vi "Subtract DAQ Offset.vi"(8 "error in (no error)":errorcluster, 11 "Instrument.DAQ":refnum<class "Instrument.DAQ.lvclass">) -> (0 "error out":errorcluster, 3 "Instrument.DAQ out":refnum<class "Instrument.DAQ.lvclass">)   [LabVIEW 2019, in "Instrument.DAQ.lvclass"]
uses:
  Instrument.DAQ.lvclass
  Instrument.DAQ.lvclass/Instrument.DAQ.ctl
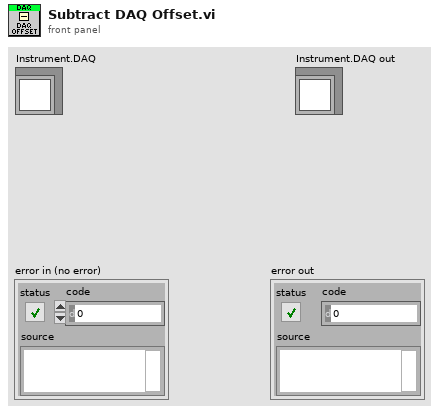
[diagram p1: front panel]
types:
  T1 = typedef "Instrument.DAQ.lvclass/Channel.Gain--Cluster--Array.ctl" = T2[]
  T2 = typedef "Instrument.DAQ.lvclass/Channel.Gain--Cluster.ctl" = cluster{"Channel":string, "Gain":dbl}
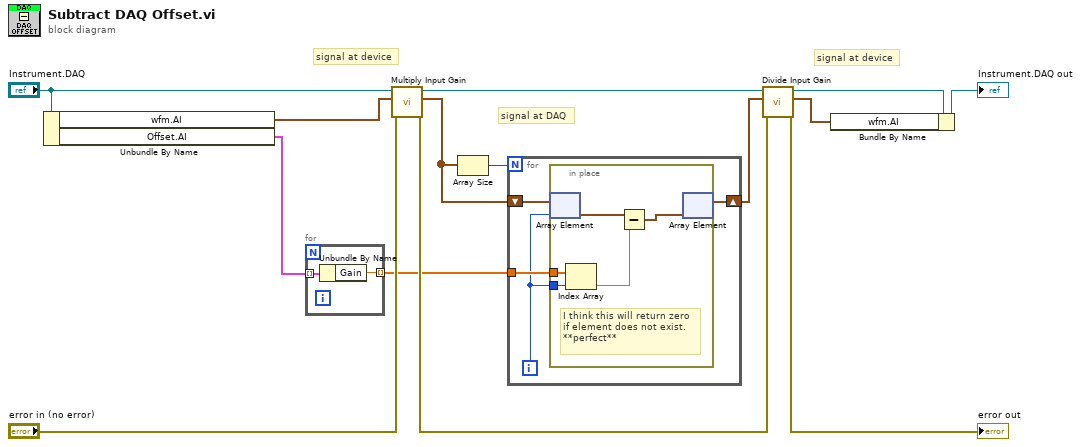
[diagram p0: block diagram]
diagram:
  # "signal at device"
  # "signal at DAQ"
  # "signal at device"
  n1 = Unbundle By Name("Instrument.DAQ") -> ("wfm.AI"=w7:waveform(dbl)[], "Offset.AI"=w4:T1)
  n2 = for {
    tunnel: w4 -> [w16] mode=indexing
    tunnel: [w15] -> w3 mode=indexing
    n3 = Unbundle By Name(w16) -> ("Gain"=w15:dbl)
  }
  n4 = call "Multiply Input Gain.vi"("error in (no error)"="error in (no error)", "WFM in"=w7, "Instrument.DAQ"="Instrument.DAQ") -> ("error out"=w10:errorcluster, "WFM out"=w5:waveform(dbl)[], "Instrument.DAQ out"=w9:refnum<class "Instrument.DAQ.lvclass">)  [unwired: 6 in]
  n5 = Array Size(array=w5) -> (size(s)=w14:i32)
  n6 = for {
    N: w14 -> [_]
    tunnel: w3 -> [w20]
    shift-right: [w17] -> w13
    shift-left: w5 -> [w18]
    i -> [w19]
    n7 = in-place {
      in-place-border: w19 -> [w25]
      in-place-border: w20 -> [w24]
      # "I think this will return zero\nif element does not exist.\n**perfect**"
      n8 = in-place-array #1(w18, w19) -> (w21:waveform(dbl))
      n9 = Index Array(array=w24, index=w25) -> (element=w23:dbl)
      n10 = Subtract(x=w21, y=w23) -> (x-y=w22:waveform(dbl))
      n11 = in-place-array #1(w22) -> (w17:waveform(dbl)[])  [unwired: 1 out]
    }
  }
  n12 = call "Divide Input Gain.vi"("error in (no error)"=w10, "WFM in"=w13, "Instrument.DAQ"=w9) -> ("error out"=→"error out":errorcluster, "WFM out"=w1:waveform(dbl)[], "Instrument.DAQ out"=w6:refnum<class "Instrument.DAQ.lvclass">)  [unwired: 6 in]
  n13 = Bundle By Name(cluster=w6, "wfm.AI"=w1) -> (→"Instrument.DAQ out":refnum<class "Instrument.DAQ.lvclass">)
